vi "Read Message.vi"(8 "error in (no error)":errorcluster, 11 "Debug Data in":refnum<class "Debug Data.lvclass">) -> (0 "error out":errorcluster, 1 "Message Data":variant, 2 "Message":string, 3 "Debug Data out":refnum<class "Debug Data.lvclass">)   [LabVIEW 2020, in "Debug Data.lvclass"]
uses:
  Debug Data.lvclass
  Debug Data.lvclass/Debug Data.ctl
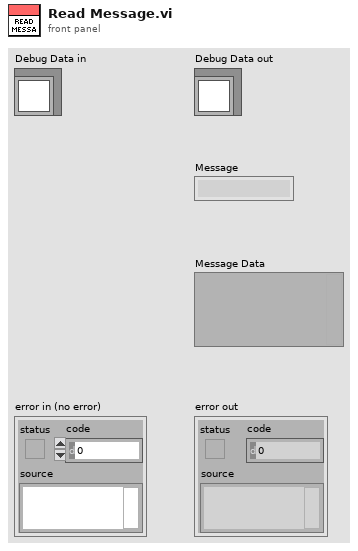
[diagram p1: front panel]
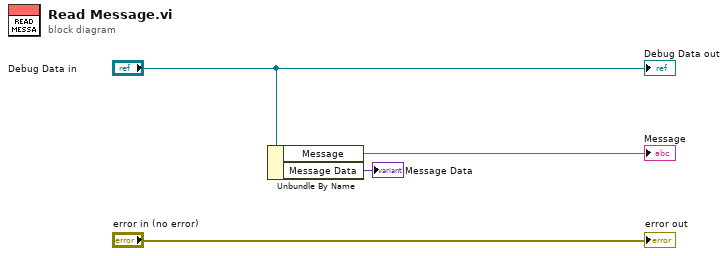
[diagram p0: block diagram]
diagram:
  n1 = Unbundle By Name("Debug Data in") -> ("Message"=→"Message":string, "Message Data"=→"Message Data":variant)
  "error out" <- "error in (no error)"
  "Debug Data out" <- "Debug Data in"
